vi "Test-Log Status.vi"(8 "error in":errorcluster, 10 "Event Data String":string, 11 "Event String":string) -> (0 "error out":errorcluster)   [LabVIEW 2017]
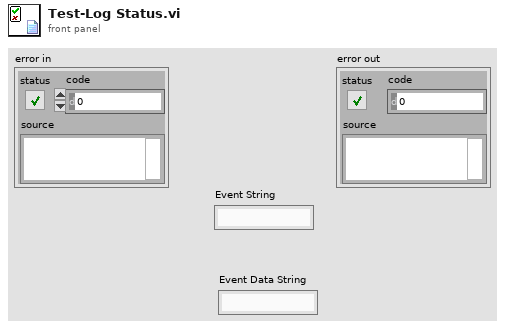
[diagram p1: front panel]
types:
  T1 = enum16{"open", "replace", "create", "open or create", "replace or create", "replace or create with confirmation"}
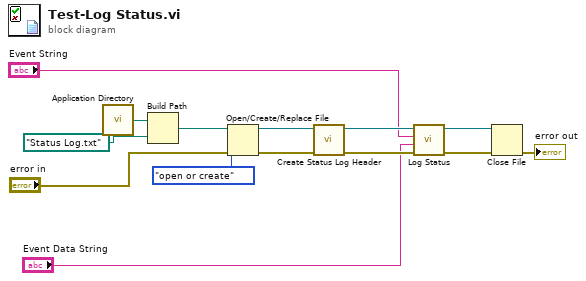
[diagram p0: block diagram]
diagram:
  n1 = call <vilib>:"Application Directory.vi"() -> ("Application Directory"=w14:path)
  n2 = Build Path(base path=w14, name or relative path=path "Status Log.txt") -> (appended path=w5:path)
  n3 = Open/Create/Replace File(file path (use dialog)=w5, error in="error in", operation (0:open)=T1."open or create") -> (refnum out=w11:refnum<file>, error out=w10:errorcluster)  [unwired: 3 in, 1 out]
  n4 = call "Create Status Log Header.vi"("error in"=w10, "Log File Refnum in"=w11) -> ("error out"=w8:errorcluster, "Log File Refnum out"=w9:refnum<file>)  [unwired: 8 in]
  n5 = call "Log Status.vi"("error in"=w8, "Event Data String (-)"="Event Data String", "Event String"="Event String", "Log File Refnum In"=w9) -> ("error out"=w6:errorcluster, "Log File Refnum Out"=w7:refnum<file>)  [unwired: 6 in]
  n6 = Close File(refnum=w7, error in=w6) -> (error out=→"error out":errorcluster)  [unwired: 1 out]
